vi "TimeDiff.vi"(1 "Time B":u32, 2 "Time A":u32) -> (0 "Time Diff":u32)   [LabVIEW 2015]
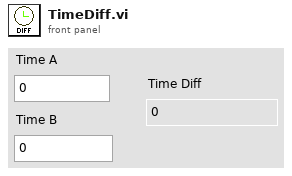
[diagram p1: front panel]
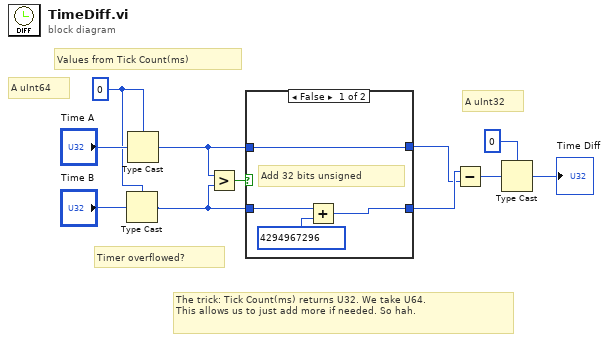
[diagram p0: block diagram]
diagram:
  w4 = u64 0
  # "A uInt32"
  # "A uInt64"
  # "Timer overflowed?"
  # "The trick: Tick Count(ms) returns U32. We take U64.\nThis allows us to just add more if needed. So hah."
  # "Values from Tick Count(ms)"
  n1 = Type Cast(type=w4, x="Time B") -> (*(type *) &x=w6:u64)
  n2 = Type Cast(type=w4, x="Time A") -> (*(type *) &x=w8:u64)
  n3 = Greater?(x=w8, y=w6) -> (0:w11:bool)
  n4 = case shown="False" w11 {
    tunnel: w6 -> [w15 w17]
    tunnel: [w13 w17] -> w10
    tunnel: [w12 w16] -> w9
    tunnel: w8 -> [w12 w16]
    frame False {
      # "Add 32 bits unsigned"
      n5 = Add(x=w15, y=u64 4294967296) -> (x+y=w13:u64)
    }
    frame True {
      # "Do nothing"
    }
  }
  n6 = Subtract(x=w10, y=w9) -> (x-y=w2:u64)
  n7 = Type Cast(type=u32 0, x=w2) -> (*(type *) &x=→"Time Diff":u32)
